vi "password.vi"(9 "Action":enum16{"Compare", "Set"}(ring), 11 "password":string) -> (3 "Success?":bool)   [LabVIEW 2013]
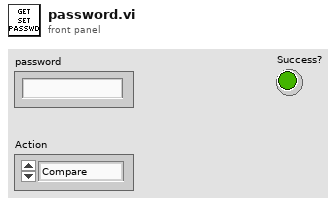
[diagram p1: front panel]
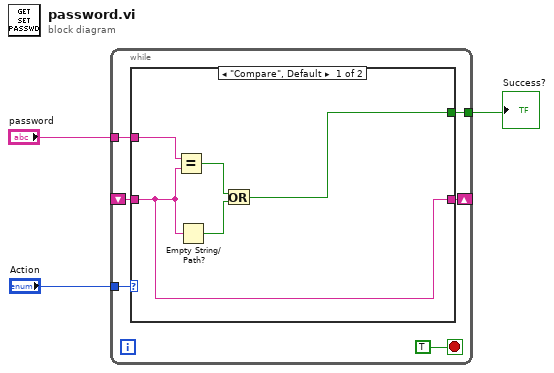
[diagram p0: block diagram]
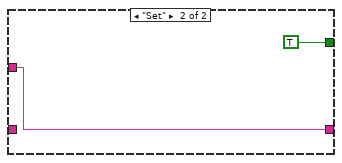
[diagram p2: hidden frame]
diagram:
  n1 = while {
    tunnel: "Action" -> [w8]
    tunnel: "password" -> [w7]
    shift-right: [w6] -> _
    shift-left: _ -> [w4]
    tunnel: [w5] -> w1
    stop <- TRUE stop-if-true
    n2 = case shown="\"Compare\", Default" w8 {
      tunnel: w7 -> [w14 w16]
      tunnel: [w10 w16] -> w6
      tunnel: [w11 TRUE] -> w5
      tunnel: w4 -> [w10 _]
      frame "Compare", Default {
        n3 = Equal?(x=w14, y=w10) -> (x = y?=w13:bool)
        n4 = Empty String/Path?(string/path=w10) -> (empty?=w12:bool)
        n5 = Or(x=w13, y=w12) -> (x .or. y?=w11:bool)
      }
      frame "Set" {
      }
    }
  }
  "Success?" <- w1
